vi "FreeCounter.vi"(4 "Reset Counter":bool caption="Reset Counter (F)") -> (1 "Counter":i32)   [LabVIEW 2017, in "GPNumeric.lvlib"]
doc: "Outputs an incrementing <B>Counter</B> when called repeatedly.\n\nThe counter starts at 1, increments by one for each consecutive call of this VI, and is latched at I32 max if it reaches that. Setting <B>Reset counter</B> to True makes <B>Counter</B> start from 1 again.\n\nThis counter is unique per instance (as it is inlined into the caller).\n\nSteen Schmidt\nGPower\n7/4 2014"
uses:
  GPNumeric.lvlib
panel:
  # "Copyright © 2016\nGPower\nSee enclosed license file for terms and conditions"
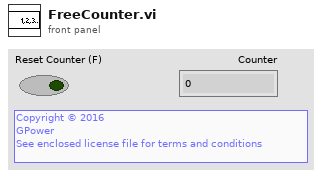
[diagram p1: front panel]
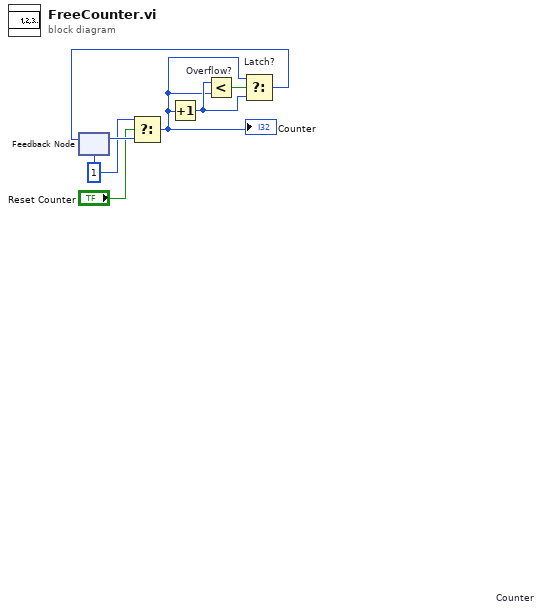
[diagram p0: block diagram]
diagram:
  w1 = 1
  n1 = feedback #1 "Counter"(w1) -> (w7:i32)
  n2 = Select(t=w1, s="Reset Counter", f=w7) -> (s? t:f=w2:i32)
  "Counter" <- w2
  n3 = Increment(x=w2) -> (x+1=w5:i32)
  n4 = Less? "Overflow?"(x=w5, y=w2) -> (x < y?=w6:bool)
  n5 = Select "Latch?"(t=w2, s=w6, f=w5) -> (s? t:f=w4:i32)
  n6 = feedback-in #1(w4) -> ()
